vi "common_errors.vi"(0 "common_errors":T1=enum."noDevices", 7 "dialog? (T)":bool=TRUE, 9 "transmit? (T)":bool=TRUE, 12 "supp_text":string[](array[string])) -> (15 "error out":errorcluster)   [LabVIEW 2020, in "common.lvlib"]
doc: "Traps and handles errors commonly seen during Performax hardware communication.\n\nProduced By:\n\n<B>Kod Integrations, LLC</B>\n4835 Marianne Drive\nMount Airy, MD 21771\nhttp://www.kodintegrations.com\nemail: info@kodintegrations.com\nphone: (240) 687-1288"
uses:
  common.lvlib
  error_actions.ctl
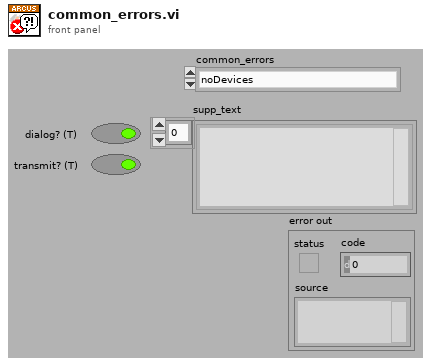
[diagram p1: front panel]
types:
  T1 = typedef "common.lvlib/error_actions.ctl" = enum16{"clearBuff", "closeRef", "nodeErr", "noDeviceInfo", "noDevices", "openRef", "sendReceive", "setTimeouts", "unknown"}
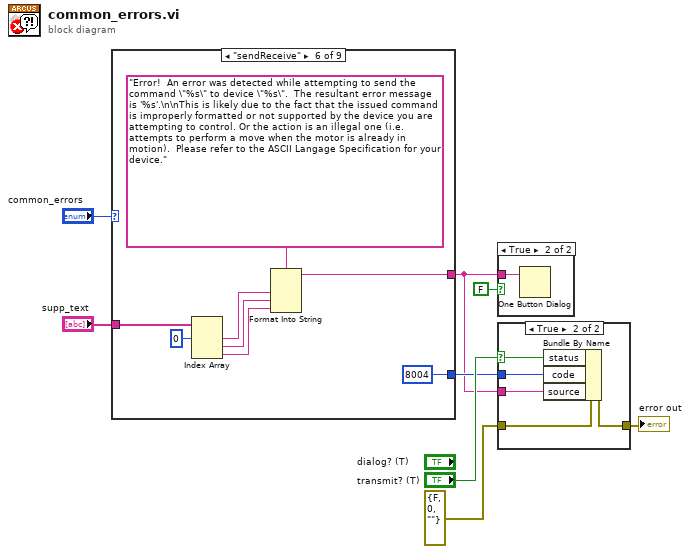
[diagram p0: block diagram]
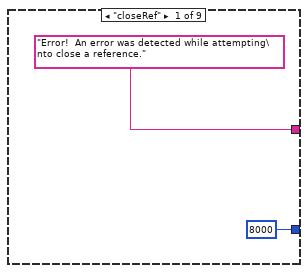
[diagram p4: hidden frame]
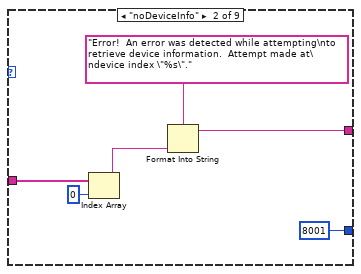
[diagram p5: hidden frame]
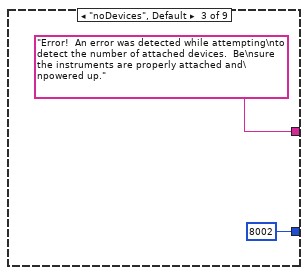
[diagram p6: hidden frame]
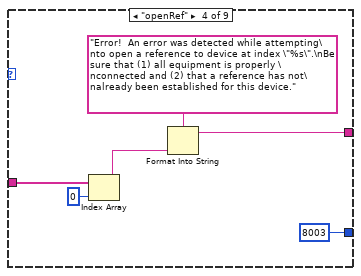
[diagram p7: hidden frame]
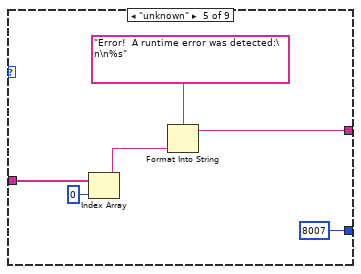
[diagram p8: hidden frame]
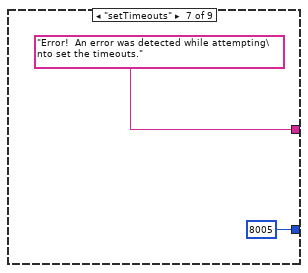
[diagram p9: hidden frame]
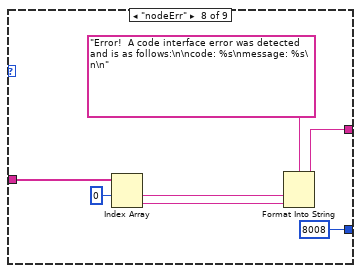
[diagram p10: hidden frame]
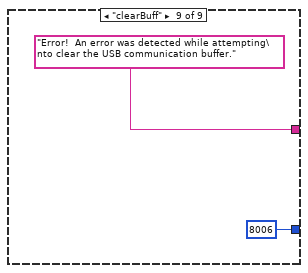
[diagram p11: hidden frame]
diagram:
  n1 = case shown="\"sendReceive\"" "common_errors" {
    tunnel: ["Error!  An error was detected while attempting\nto close a reference." w12 "Error!  An error was detected while attempting\nto detect the number of attached devices.  Be\nsure the instruments are properly attached and\npowered up." w20 w26 w34 "Error!  An error was detected while attempting\nto set the timeouts." w41 "Error!  An error was detected while attempting\nto clear the USB communication buffer."] -> w3
    tunnel: [8000 8001 8002 8003 8007 8004 8005 8008 8006] -> w6
    tunnel: "supp_text" -> [_ w15 _ w23 w29 w37 _ w44 _]
    frame "closeRef" {
    }
    frame "noDeviceInfo" {
      n2 = Index Array(array=w15, index=0) -> (element=w13:string)
      n3 = Format Into String(format string="Error!  An error was detected while attempting\nto retrieve device information.  Attempt made at\ndevice index \"%s\".", w13) -> (resulting string=w12:string)  [unwired: 2 in, 1 out]
    }
    frame "noDevices", Default {
    }
    frame "openRef" {
      n4 = Index Array(array=w23, index=0) -> (element=w21:string)
      n5 = Format Into String(format string="Error!  An error was detected while attempting\nto open a reference to device at index \"%s\".\nBe sure that (1) all equipment is properly \nconnected and (2) that a reference has not\nalready been established for this device.", w21) -> (resulting string=w20:string)  [unwired: 2 in, 1 out]
    }
    frame "unknown" {
      n6 = Index Array(array=w29, index=0) -> (element=w27:string)
      n7 = Format Into String(format string="Error!  A runtime error was detected:\n\n%s", w27) -> (resulting string=w26:string)  [unwired: 2 in, 1 out]
    }
    frame "sendReceive" {
      n8 = Index Array(array=w37, index #1=0 ("index")) -> (element #1=w35:string, element #2=w32:string, element #3=w31:string)  [unwired: 2 in]
      n9 = Format Into String(format string="Error!  An error was detected while attempting to send the command \"%s\" to device \"%s\".  The resultant error message is '%s'.\n\nThis is likely due to the fact that the issued command is improperly formatted or not supported by the device you are attempting to control. Or the action is an illegal one (i.e. attempts to perform a move when the motor is already in motion).  Please refer to the ASCII Langage Specification for your device.", w35, w32, w31) -> (resulting string=w34:string)  [unwired: 2 in, 1 out]
    }
    frame "setTimeouts" {
    }
    frame "nodeErr" {
      n10 = Index Array(array=w44, index #1=0 ("index")) -> (element #1=w43:string, element #2=w42:string)  [unwired: 1 in]
      n11 = Format Into String(format string="Error!  A code interface error was detected and is as follows:\n\ncode: %s\nmessage: %s\n\n", w43, w42) -> (resulting string=w41:string)  [unwired: 2 in, 1 out]
    }
    frame "clearBuff" {
    }
  }
  n12 = case shown="True" FALSE {
    tunnel: w3 -> [_ w50]
    frame False {
    }
    frame True {
      n13 = One Button Dialog(message=w50) -> ()  [unwired: 1 in, 1 out]
    }
  }
  n14 = case shown="True" "transmit? (T)" {
    selector: "transmit? (T)" -> [_ w53]
    tunnel: errorcluster {"status"=FALSE, "code"=0, "source"=""} ("error out") -> [w51 w56]
    tunnel: w6 -> [_ w55]
    tunnel: w3 -> [_ w54]
    tunnel: [w51 w52] -> w5
    frame False {
    }
    frame True {
      n15 = Bundle By Name(cluster=w56, "status"=w53, "code"=w55, "source"=w54) -> (w52:errorcluster)
    }
  }
  "error out" <- w5
